vi "ClassDiagramGraph_Create.vi"(0 "reference":refnum<class "ClassDiagramGraph.lvclass">, 5 "error in (no error)":errorcluster) -> (14 "reference out":refnum<class "ClassDiagramGraph.lvclass">, 19 "error out":errorcluster)   [LabVIEW 2014, in "ClassDiagramGraph.lvclass"]
doc: "Creates and initializes a new ClassDiagramGraph object.\n\nThis object should be destroyed using a ClassDiagramGraph destructor VI or a virtual base class destructor VI.\n\n[GOOP 2.1]"
uses:
  <resource>/Framework/Providers/Open_GDS/UML/ClassDiagramGraph_class/ClassDiagramGraph.lvclass
  <resource>/Framework/Providers/Open_GDS/UML/ArrowHead_class/ArrowHeadType.ctl
  <resource>/Framework/Providers/Open_GDS/UML/BentStyle_class/BentStyleType.ctl
  <resource>/Framework/Providers/Open_GDS/UML/UMLEditor/UMLEditor toolsType.ctl
  <resource>/Framework/Providers/Open_GDS/UML/LineStyle_class/LineStyleType.ctl
  <resource>/Framework/Providers/Open_GDS/UML/Graphics_class/StrokeType.ctl
  <resource>/Framework/Providers/Open_GDS/UML/ClassRelationshipEdge_class/ClassRelationshipEdge.lvclass
  <resource>/Framework/Providers/Open_GDS/UML/Graph_class/Graph.lvclass
  <resource>/Framework/Providers/Open_GDS/UML/ClassNode_class/ClassNode.lvclass
  <resource>/Framework/Providers/Open_GDS/UML/InterfaceNode_class/InterfaceNode.lvclass
  <resource>/Framework/Providers/Open_GDS/UML/NoteNode_class/NoteNode.lvclass
  <resource>/Framework/Providers/Open_GDS/UML/PackageNode_class/PackageNode.lvclass
  <resource>/Framework/Providers/Open_GDS/UML/ArrowHead_class/ArrowHead.lvclass
  <resource>/Framework/Providers/Open_GDS/UML/BentStyle_class/BentStyle.lvclass
  <resource>/Framework/Providers/Open_GDS/UML/SegmentedLineEdge_class/SegmentedLineEdge.lvclass
  <resource>/Framework/Providers/Open_GDS/UML/NoteEdge_class/NoteEdge.lvclass
  <resource>/Framework/Providers/Open_GDS/UML/Graphics_class/Graphics.lvclass
  <resource>/Framework/Providers/Open_GDS/UML/LineStyle_class/LineStyle.lvclass
panel:
  # "The input reference should only\nbe wired when this method is called\nby a sub class constructor."
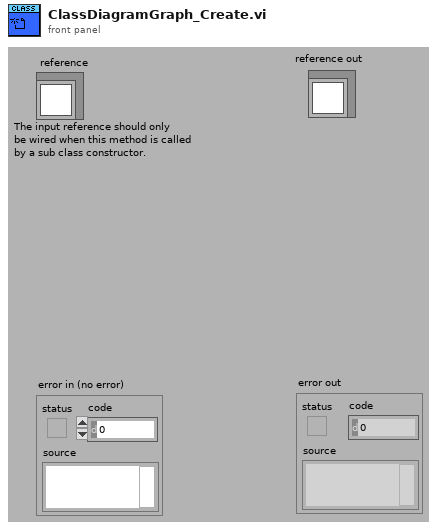
[diagram p1: front panel]
types:
  T1 = typedef "LineStyle.lvclass/LineStyleType.ctl" = enum16{"SOLID", "DOTTED"}
  T2 = typedef "UMLEditor toolsType.ctl" = enum16{"CD_Select", "CD_Class", "CD_Interface", "CD_Package", "CD_Note", "CD_Dependency", "CD_Inheritance", "CD_InterfaceImp", "CD_Association", "CD_Aggregation", "CD_Composite", "CD_NoteConn", "SQD_Select", "SQD_Object", "SQD_ActionBar", "SQD_Note", "SQD_Call", "SQD_NoteConn", "UD_Select", "UD_System", "UD_Actor", "UD_UseCase", "UD_Note", "UD_Assoiciation", "UD_Generalization", "UD_GeneralizationIncludes", "UD_GeneralizationExtends", "UD_Realization", "UD_Relationship", "UD_NoteEdge", "STD_Select", "STD_State", "STD_InitailState", "STD_FinalState", "STD_ChoiseState", "STD_StateTransation", "STD_Note", "STD_NoteEdge", "DM_Select", "DM_VI", "DM_Module", "DM_Request", "DM_RequestWait", "DM_Roundtrip", "DM_Broadcast", "DM_Note", "DM_NoteEdge"}
  T3 = typedef "BentStyle.lvclass/BentStyleType.ctl" = enum16{"STRAIGHT", "HV", "VH", "HVH", "VHV", "ARC"}
  T4 = typedef "ArrowHead.lvclass/ArrowHeadType.ctl" = enum16{"NONE", "TRIANGLE", "BLACK_TRIANGLE", "V", "HALF_V", "DIAMOND", "BLACK_DIAMOND"}
  T5 = typedef "Graphics.lvclass/StrokeType.ctl" = enum16{"USE_DEFAULT", "SOLID", "DOTTED"}
  T6 = typedef "Graph.lvclass/ClassAttributes.ctl" = cluster{"NODE_PROT":refnum<class "AbstractNode.lvclass">[], "NodeNames":string[], "EDGE_PROT":refnum<class "AbstractEdge.lvclass">[], "EdgeNames":string[]}
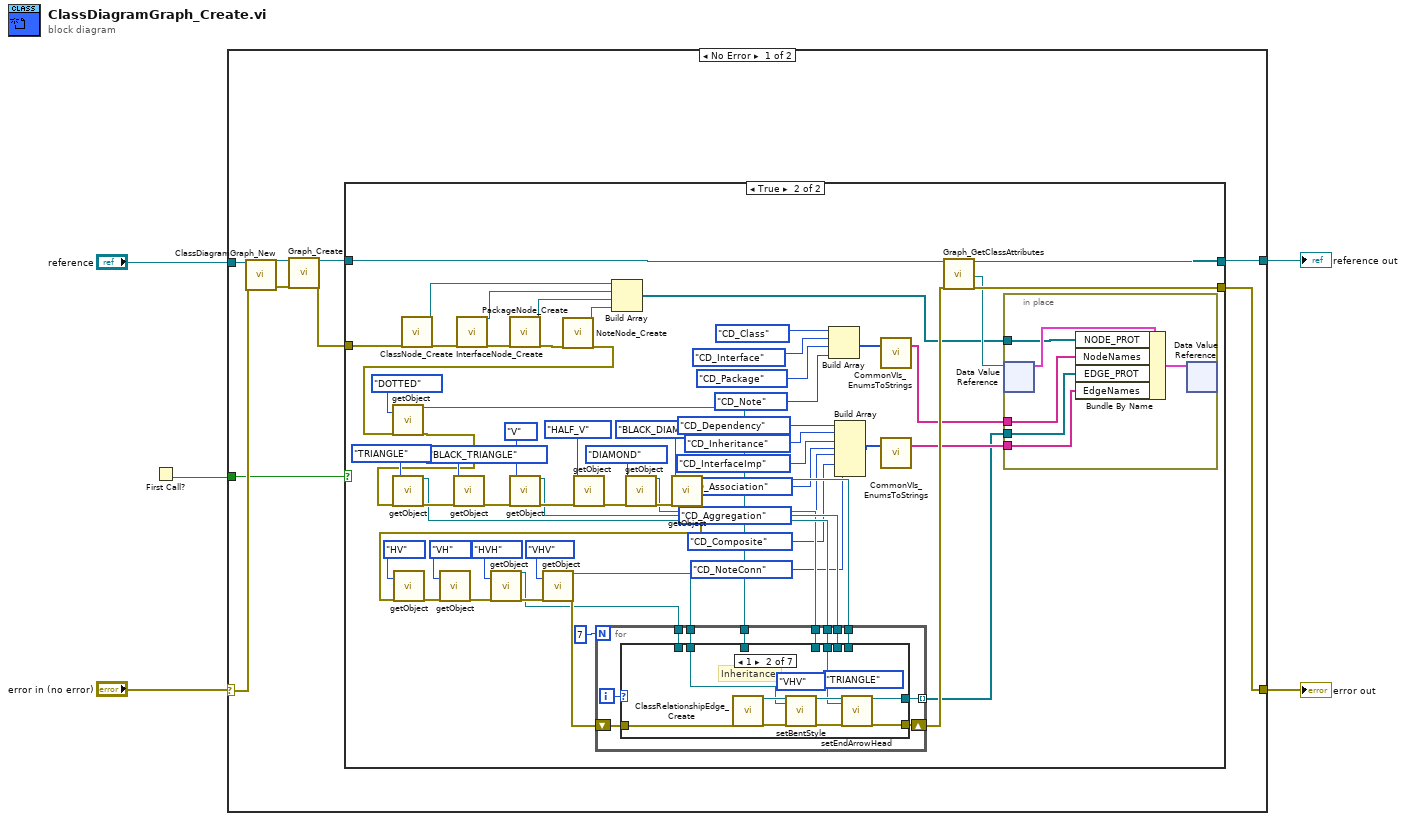
[diagram p0: block diagram]
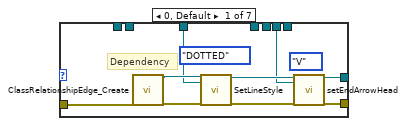
[diagram p3: hidden frame]
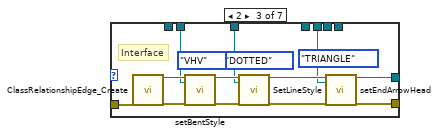
[diagram p4: hidden frame]
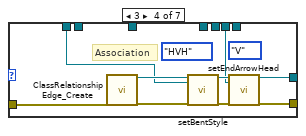
[diagram p5: hidden frame]
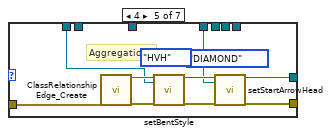
[diagram p6: hidden frame]
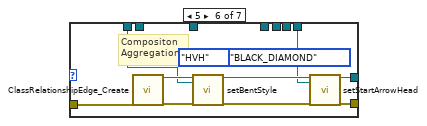
[diagram p7: hidden frame]
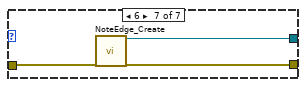
[diagram p8: hidden frame]
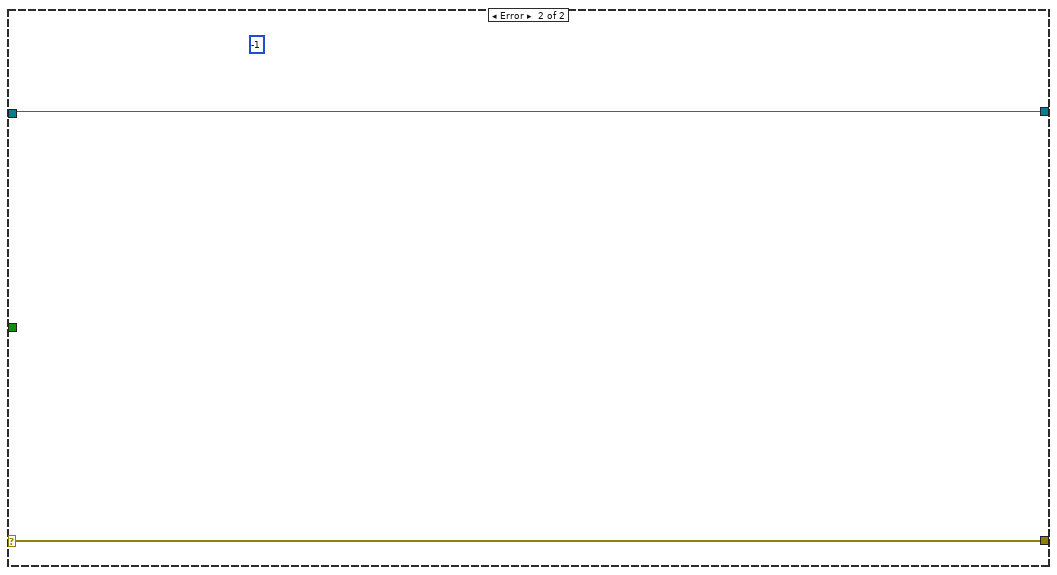
[diagram p9: hidden frame]
diagram:
  n1 = First Call?() -> (First Call?: T/F=w1:bool)
  n2 = case shown="No Error" "error in (no error)" {
    selector: "error in (no error)" -> [w14 w156]
    tunnel: [w10 w155] -> w5
    tunnel: [w9 w156] -> w4
    tunnel: "reference" -> [w13 w155]
    tunnel: w1 -> [w6 _]
    frame No Error {
      n3 = call <resource>:"ClassDiagramGraph_New.vi"("reference in"=w13, "error in (no error)"=w14) -> ("reference out"=w12:refnum<class "ClassDiagramGraph.lvclass">, "error out"=w8:errorcluster)  [unwired: 2 in, 14 out]
      n4 = call <resource>:"Graph_Create.vi"("reference"=w12, "error in (no error)"=w8) -> ("reference out"=w11:refnum<class "ClassDiagramGraph.lvclass">, "error out"=w7:errorcluster)  [unwired: 1 in, 15 out]
      n5 = case shown="True" w6 {
        tunnel: w11 -> [w16 w77]
        tunnel: [w15 w76] -> w9
        tunnel: [w16 w75] -> w10
        tunnel: w7 -> [w15 w36]
        frame False {
        }
        frame True {
          n6 = call <resource>:"ClassNode_Create.vi"("error in (no error)"=w36) -> ("reference out"=w70:refnum<class "ClassNode.lvclass">, "error out"=w73:errorcluster)  [unwired: 1 in, 16 out]
          n7 = call <resource>:"InterfaceNode_Create.vi"("error in (no error)"=w73) -> ("reference out"=w69:refnum<class "InterfaceNode.lvclass">, "error out"=w72:errorcluster)  [unwired: 1 in, 16 out]
          n8 = call <resource>:"PackageNode_Create.vi"("error in (no error)"=w72) -> ("reference out"=w68:refnum<class "PackageNode.lvclass">, "error out"=w71:errorcluster)  [unwired: 1 in, 16 out]
          n9 = call <resource>:"NoteNode_Create.vi"("error in (no error)"=w71) -> ("reference out"=w67:refnum<class "NoteNode.lvclass">, "error out"=w45:errorcluster)  [unwired: 1 in, 16 out]
          n10 = call <resource>:"getObject.vi"("lineStyle"=LineStyleType."DOTTED", "error in (no error)"=w45) -> ("reference out"=w43:refnum<class "LineStyle.lvclass">, "error out"=w54:errorcluster)  [unwired: 16 out]
          n11 = call <resource>:"getObject.vi"("arrowHead"=ArrowHeadType."TRIANGLE", "error in (no error)"=w54) -> ("reference out"=w42:refnum<class "ArrowHead.lvclass">, "error out"=w64:errorcluster)  [unwired: 16 out]
          n12 = call <resource>:"getObject.vi"("arrowHead"=ArrowHeadType."BLACK_TRIANGLE", "error in (no error)"=w64) -> ("error out"=w63:errorcluster)  [unwired: 17 out]
          n13 = call <resource>:"getObject.vi"("arrowHead"=ArrowHeadType."V", "error in (no error)"=w63) -> ("reference out"=w40:refnum<class "ArrowHead.lvclass">, "error out"=w60:errorcluster)  [unwired: 16 out]
          n14 = call <resource>:"getObject.vi"("arrowHead"=ArrowHeadType."HALF_V", "error in (no error)"=w60) -> ("error out"=w58:errorcluster)  [unwired: 17 out]
          n15 = Build Array(w70, w69, w68, w67) -> (w21:refnum<class "RectangularNode.lvclass">[])
          n16 = call <resource>:"getObject.vi"("arrowHead"=ArrowHeadType."DIAMOND", "error in (no error)"=w58) -> ("reference out"=w38:refnum<class "ArrowHead.lvclass">, "error out"=w56:errorcluster)  [unwired: 16 out]
          n17 = call <resource>:"getObject.vi"("arrowHead"=ArrowHeadType."BLACK_DIAMOND", "error in (no error)"=w56) -> ("reference out"=w37:refnum<class "ArrowHead.lvclass">, "error out"=w53:errorcluster)  [unwired: 16 out]
          n18 = call <resource>:"getObject.vi"("bentStyle"=BentStyleType."HV", "error in (no error)"=w53) -> ("error out"=w48:errorcluster)  [unwired: 17 out]
          n19 = call <resource>:"getObject.vi"("bentStyle"=BentStyleType."VH", "error in (no error)"=w48) -> ("error out"=w47:errorcluster)  [unwired: 17 out]
          n20 = call <resource>:"getObject.vi"("bentStyle"=BentStyleType."HVH", "error in (no error)"=w47) -> ("reference out"=w39:refnum<class "BentStyle.lvclass">, "error out"=w46:errorcluster)  [unwired: 16 out]
          n21 = call <resource>:"getObject.vi"("bentStyle"=BentStyleType."VHV", "error in (no error)"=w46) -> ("reference out"=w44:refnum<class "BentStyle.lvclass">, "error out"=w41:errorcluster)  [unwired: 16 out]
          n22 = for {
            N: 7 -> [_]
            shift-right: [w91] -> w66
            shift-left: w41 -> [w93]
            tunnel: [w92] -> w18 mode=indexing
            tunnel: w44 -> [w90]
            tunnel: w43 -> [w89]
            tunnel: w42 -> [w88]
            tunnel: w40 -> [w87]
            tunnel: w39 -> [w86]
            tunnel: w38 -> [w85]
            tunnel: w37 -> [w84]
            i -> [w94]
            n23 = case shown="1" w94 {
              tunnel: w93 -> [w103 w112 w124 w133 w142 w151 w152]
              tunnel: [w98 w109 w123 w132 w141 w150 w154] -> w92
              tunnel: [w97 w108 w122 w131 w136 w145 w153] -> w91
              tunnel: w90 -> [_ w105 w115 _ _ _ _]
              tunnel: w89 -> [w96 _ w114 _ _ _ _]
              tunnel: w88 -> [_ w104 w113 _ _ _ _]
              tunnel: w87 -> [w95 _ _ w125 _ _ _]
              tunnel: w86 -> [_ _ _ w126 w135 w144 _]
              tunnel: w85 -> [_ _ _ _ w134 _ _]
              tunnel: w84 -> [_ _ _ _ _ w143 _]
              frame 0, Default {
                (unwired) ArrowHeadType."V" ("arrowHead")
                (unwired) StrokeType."DOTTED" ("lineStyle")
                # "Dependency"
                n24 = call <resource>:"ClassRelationshipEdge_Create.vi"("error in (no error)"=w103) -> ("reference out"=w102:refnum<class "ClassRelationshipEdge.lvclass">, "error out"=w101:errorcluster)  [unwired: 1 in, 16 out]
                n25 = call-dynamic "SetLineStyle.vi"("reference"=w102, "lineStyle"=w96, "error in (no error)"=w101) -> ("reference out"=w100:refnum<class "ClassRelationshipEdge.lvclass">, "error out"=w99:errorcluster)  [unwired: 15 in]
                n26 = call-dynamic "setEndArrowHead.vi"("reference"=w100, "endArrowHead"=w95, "error in (no error)"=w99) -> ("reference out"=w98:refnum<class "ClassRelationshipEdge.lvclass">, "error out"=w97:errorcluster)  [unwired: 15 in]
              }
              frame 1 {
                (unwired) BentStyleType."VHV" ("bentStyle")
                (unwired) ArrowHeadType."TRIANGLE" ("arrowHead")
                # "Inheritance"
                n27 = call <resource>:"ClassRelationshipEdge_Create.vi"("error in (no error)"=w112) -> ("reference out"=w107:refnum<class "ClassRelationshipEdge.lvclass">, "error out"=w106:errorcluster)  [unwired: 1 in, 16 out]
                n28 = call <resource>:"setBentStyle.vi"("reference"=w107, "newBentStyle"=w105, "error in (no error)"=w106) -> ("reference out"=w111:refnum<class "ClassRelationshipEdge.lvclass">, "error out"=w110:errorcluster)  [unwired: 15 out]
                n29 = call-dynamic "setEndArrowHead.vi"("reference"=w111, "endArrowHead"=w104, "error in (no error)"=w110) -> ("reference out"=w109:refnum<class "ClassRelationshipEdge.lvclass">, "error out"=w108:errorcluster)  [unwired: 15 in]
              }
              frame 2 {
                (unwired) StrokeType."DOTTED" ("lineStyle")
                (unwired) BentStyleType."VHV" ("bentStyle")
                (unwired) ArrowHeadType."TRIANGLE" ("arrowHead")
                # "Interface"
                n30 = call <resource>:"ClassRelationshipEdge_Create.vi"("error in (no error)"=w124) -> ("reference out"=w121:refnum<class "ClassRelationshipEdge.lvclass">, "error out"=w120:errorcluster)  [unwired: 1 in, 16 out]
                n31 = call <resource>:"setBentStyle.vi"("reference"=w121, "newBentStyle"=w115, "error in (no error)"=w120) -> ("reference out"=w119:refnum<class "ClassRelationshipEdge.lvclass">, "error out"=w118:errorcluster)  [unwired: 15 out]
                n32 = call-dynamic "SetLineStyle.vi"("reference"=w119, "lineStyle"=w114, "error in (no error)"=w118) -> ("reference out"=w117:refnum<class "ClassRelationshipEdge.lvclass">, "error out"=w116:errorcluster)  [unwired: 15 in]
                n33 = call-dynamic "setEndArrowHead.vi"("reference"=w117, "endArrowHead"=w113, "error in (no error)"=w116) -> ("reference out"=w123:refnum<class "ClassRelationshipEdge.lvclass">, "error out"=w122:errorcluster)  [unwired: 15 in]
              }
              frame 3 {
                (unwired) BentStyleType."HVH" ("bentStyle")
                (unwired) ArrowHeadType."V" ("arrowHead")
                # "Association"
                n34 = call <resource>:"ClassRelationshipEdge_Create.vi"("error in (no error)"=w133) -> ("reference out"=w130:refnum<class "ClassRelationshipEdge.lvclass">, "error out"=w129:errorcluster)  [unwired: 1 in, 16 out]
                n35 = call <resource>:"setBentStyle.vi"("reference"=w130, "newBentStyle"=w126, "error in (no error)"=w129) -> ("reference out"=w128:refnum<class "ClassRelationshipEdge.lvclass">, "error out"=w127:errorcluster)  [unwired: 15 out]
                n36 = call-dynamic "setEndArrowHead.vi"("reference"=w128, "endArrowHead"=w125, "error in (no error)"=w127) -> ("reference out"=w132:refnum<class "ClassRelationshipEdge.lvclass">, "error out"=w131:errorcluster)  [unwired: 15 in]
              }
              frame 4 {
                (unwired) ArrowHeadType."DIAMOND" ("arrowHead")
                (unwired) BentStyleType."HVH" ("bentStyle")
                # "Aggregation"
                n37 = call <resource>:"ClassRelationshipEdge_Create.vi"("error in (no error)"=w142) -> ("reference out"=w140:refnum<class "ClassRelationshipEdge.lvclass">, "error out"=w139:errorcluster)  [unwired: 1 in, 16 out]
                n38 = call <resource>:"setBentStyle.vi"("reference"=w140, "newBentStyle"=w135, "error in (no error)"=w139) -> ("reference out"=w138:refnum<class "ClassRelationshipEdge.lvclass">, "error out"=w137:errorcluster)  [unwired: 15 out]
                n39 = call <resource>:"setStartArrowHead.vi"("reference"=w138, "arroeHead"=w134, "error in (no error)"=w137) -> ("reference out"=w141:refnum<class "ClassRelationshipEdge.lvclass">, "error out"=w136:errorcluster)  [unwired: 15 out]
              }
              frame 5 {
                (unwired) ArrowHeadType."BLACK_DIAMOND" ("arrowHead")
                (unwired) BentStyleType."HVH" ("bentStyle")
                # "Compositon\nAggregation"
                n40 = call <resource>:"ClassRelationshipEdge_Create.vi"("error in (no error)"=w151) -> ("reference out"=w149:refnum<class "ClassRelationshipEdge.lvclass">, "error out"=w148:errorcluster)  [unwired: 1 in, 16 out]
                n41 = call <resource>:"setBentStyle.vi"("reference"=w149, "newBentStyle"=w144, "error in (no error)"=w148) -> ("reference out"=w147:refnum<class "ClassRelationshipEdge.lvclass">, "error out"=w146:errorcluster)  [unwired: 15 out]
                n42 = call <resource>:"setStartArrowHead.vi"("reference"=w147, "arroeHead"=w143, "error in (no error)"=w146) -> ("reference out"=w150:refnum<class "ClassRelationshipEdge.lvclass">, "error out"=w145:errorcluster)  [unwired: 15 out]
              }
              frame 6 {
                n43 = call <resource>:"NoteEdge_Create.vi"("error in (no error)"=w152) -> ("reference out"=w154:refnum<class "NoteEdge.lvclass">, "error out"=w153:errorcluster)  [unwired: 1 in, 16 out]
              }
            }
          }
          n44 = Build Array(UMLEditor_toolsType."CD_Class" ("tool"), UMLEditor_toolsType."CD_Interface" ("tool"), UMLEditor_toolsType."CD_Package" ("tool"), UMLEditor_toolsType."CD_Note" ("tool")) -> (w35:T2[])
          n45 = Build Array(UMLEditor_toolsType."CD_Dependency" ("tool"), UMLEditor_toolsType."CD_Inheritance" ("tool"), UMLEditor_toolsType."CD_InterfaceImp" ("tool"), UMLEditor_toolsType."CD_Association" ("tool"), UMLEditor_toolsType."CD_Aggregation" ("tool"), UMLEditor_toolsType."CD_Composite" ("tool"), UMLEditor_toolsType."CD_NoteConn" ("tool")) -> (w17:T2[])
          n46 = call <resource>:"CommonVIs_EnumsToStrings.vi"("ArrayEnumVariantIn"=w35) -> ("EnumItems(string)"=w20:string[])  [unwired: 2 in, 16 out]
          n47 = call <resource>:"CommonVIs_EnumsToStrings.vi"("ArrayEnumVariantIn"=w17) -> ("EnumItems(string)"=w19:string[])  [unwired: 2 in, 16 out]
          n48 = call <resource>:"Graph_GetClassAttributes.vi"("reference in"=w77, "error in (no error)"=w66) -> ("reference out"=w75:refnum<class "ClassDiagramGraph.lvclass">, "Class attribute Reference"=w22:refnum<data-value>, "error out"=w76:errorcluster)  [unwired: 14 in, 1 out]
          n49 = in-place {
            in-place-border: w21 -> [w82]
            in-place-border: w20 -> [w81]
            in-place-border: w18 -> [w80]
            in-place-border: w19 -> [w79]
            n50 = in-place-dvr #1(w22) -> (w83:T6)  [unwired: 1 out]
            n51 = Bundle By Name(cluster=w83, "NODE_PROT"=w82, "NodeNames"=w81, "EDGE_PROT"=w80, "EdgeNames"=w79) -> (w78:T6)
            n52 = in-place-dvr #1(w78) -> ()  [unwired: 2 out]
          }
        }
      }
    }
    frame Error {
      (unwired) -1 ("Nr of open handles")
    }
  }
  "error out" <- w4
  "reference out" <- w5
